vi "3 - Dado.vi"() -> ()   [LabVIEW 2020]
uses:
  <vilib>/numeric/Random Number (Range) U64.vi
  <vilib>/numeric/sub_Random U32.vi
panel:
  out "Tentativas":dbl
  in  "Dado 2":dbl
  in  "Dado 1":dbl
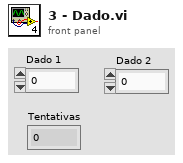
[diagram p1: front panel]
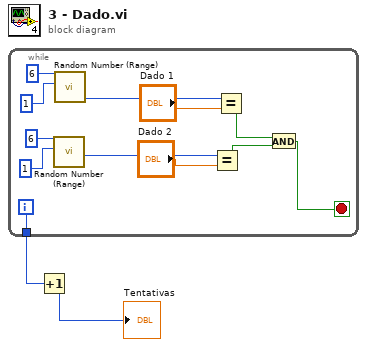
[diagram p0: block diagram]
diagram:
  n1 = while {
    tunnel: [w3] -> w1
    i -> [w3]
    stop <- w4 stop-if-true
    n2 = call-poly <vilib>:"Random Number (Range).vi"("lower bound (0)"=1, "upper bound (100)"=6) -> ("number"=w6:u64)  [unwired: 9 in]
    n3 = call-poly <vilib>:"Random Number (Range).vi"("lower bound (0)"=1, "upper bound (100)"=6) -> ("number"=w7:u64)  [unwired: 9 in]
    n4 = Equal?(x=w6, y="Dado 2") -> (x = y?=w9:bool)
    n5 = Equal?(x=w7, y="Dado 1") -> (x = y?=w10:bool)
    n6 = And(x=w10, y=w9) -> (x .and. y?=w4:bool)
  }
  n7 = Increment(x=w1) -> (x+1=→"Tentativas":i32)
